vi "Set Local IP Address.vi"(10 "Local IP Address":string, 11 "Host Reply Time Test Actor in":refnum<class "Host Reply Time Test Actor.lvclass">) -> (3 "Host Reply Time Test Actor out":refnum<class "Host Reply Time Test Actor.lvclass">)   [LabVIEW 2023, in "Host Reply Time Test Actor.lvlib" / "Host Reply Time Test Actor.lvclass"]
uses:
  Host Reply Time Test Actor.lvclass
  Host Reply Time Test Actor.lvclass/Host Reply Time Test Actor.ctl
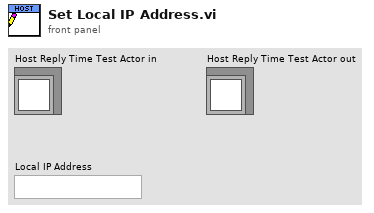
[diagram p1: front panel]
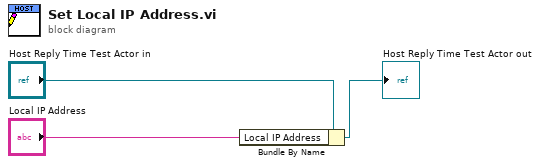
[diagram p0: block diagram]
diagram:
  n1 = Bundle By Name(cluster="Host Reply Time Test Actor in", "Local IP Address"="Local IP Address") -> (→"Host Reply Time Test Actor out":refnum<class "Host Reply Time Test Actor.lvclass">)
